vi "Release-status-notifs.vi"(8 "error in (no error)":errorcluster, 11 "Object ref in":T1) -> (0 "error out":errorcluster, 3 "Object ref out":T1)   [LabVIEW 2013, in "PowderDeposition.lvlib" / "PD-Main.lvclass"]
uses:
  PD-Main.lvclass
  Object-reference.ctl
  PD-Main.lvclass/PD-Main.ctl
  Read Abort.vi
  Read Exit.vi
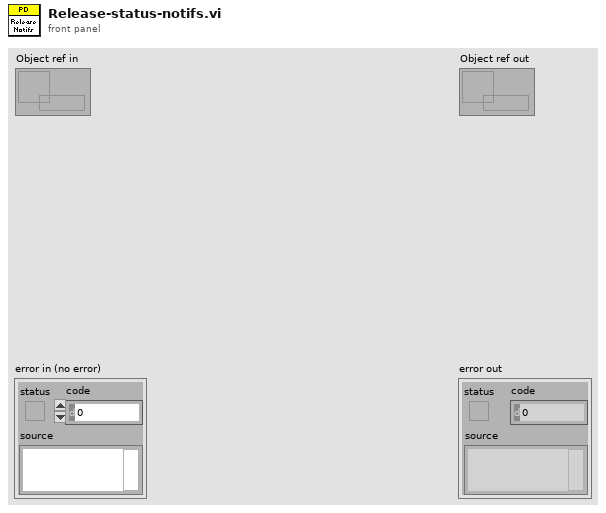
[diagram p1: front panel]
types:
  T1 = typedef "PowderDeposition.lvlib/PD-Main.lvclass/Object-reference.ctl" = refnum<data-value>
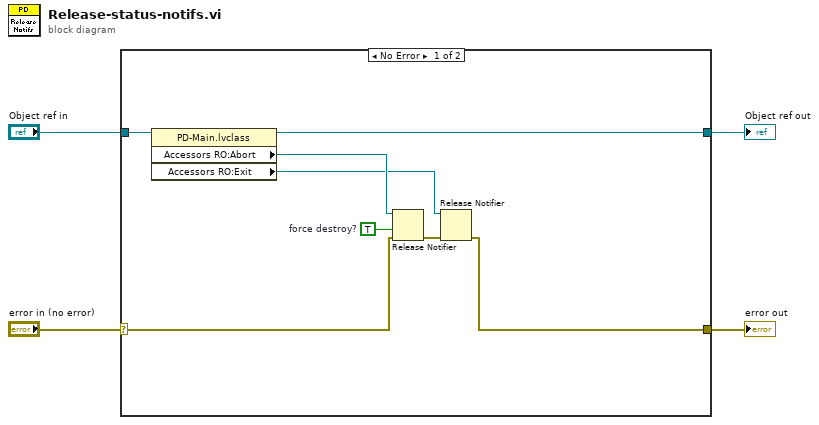
[diagram p0: block diagram]
diagram:
  n1 = case shown="No Error" "error in (no error)" {
    selector: "error in (no error)" -> [w9 w14]
    tunnel: [w6 w14] -> w3
    tunnel: [w11 w13] -> w1
    tunnel: "Object ref in" -> [w12 w13]
    frame No Error {
      w8 = TRUE  # force destroy?
      n2 = property class="PD-Main.lvclass"(reference=w12) -> (reference out=w11:T1, "Accessors RO:Abort"=w10:refnum<notifier>, "Accessors RO:Exit"=w5:refnum<notifier>)  [unwired: 1 in, 1 out]
      n3 = Release Notifier(notifier=w10, force destroy? (F)=w8, error in (no error)=w9) -> (error out=w7:errorcluster)  [unwired: 2 out]
      n4 = Release Notifier(notifier=w5, error in (no error)=w7) -> (error out=w6:errorcluster)  [unwired: 1 in, 2 out]
    }
    frame Error {
    }
  }
  "error out" <- w3
  "Object ref out" <- w1
